vi "FindAdaptableTerm.vi"(0 "Adaptable Terms":cluster{"Type":T2, "Id":T1, "Broken":bool}[](array[cluster]), 1 "Id":string) -> (2 "Type":T2, 3 "Id out":T1, 4 "Found?":bool, 5 "Broken":bool)   [LabVIEW 2017]
uses:
  <vilib>/XNodeSupport/XNodeType.ctl
  <vilib>/XNodeSupport/XNodeString.ctl
  <vilib>/XNodeSupport/NI_XNodeSupport.lvlib
panel:
  # "LVHDF5 Toolkit\nCopyright (c) 2005-2013 by Jason D. Sommerville\nCopyright (c) 2014 by UPVI, LLC.\n\nThis use and distribution of this file is governed by the terms found in \nLICENSE.txt distributed with this toolkit and installed at\n <user.lib>\\_lvhdf5\\LICENSE.txt"
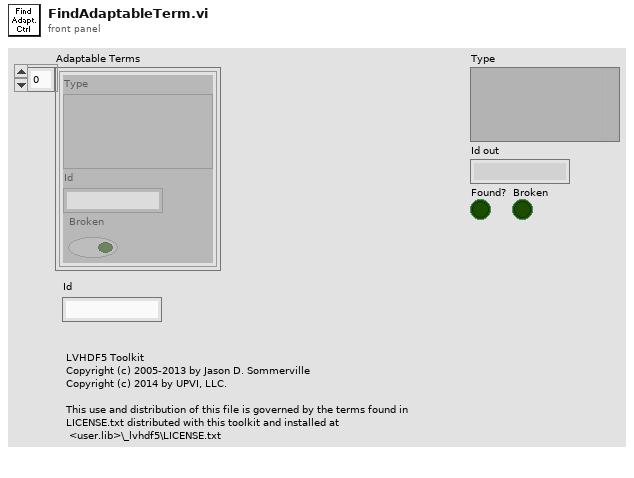
[diagram p1: front panel]
types:
  T1 = typedef "NI_XNodeSupport.lvlib/XNodeString.ctl" = string
  T2 = typedef "NI_XNodeSupport.lvlib/XNodeType.ctl" = variant
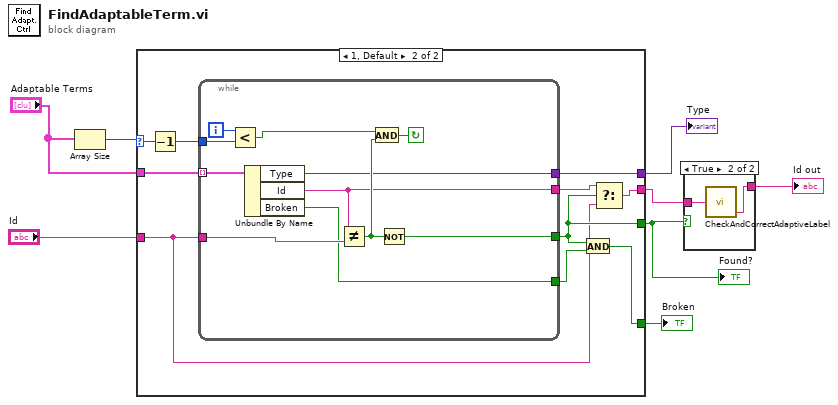
[diagram p0: block diagram]
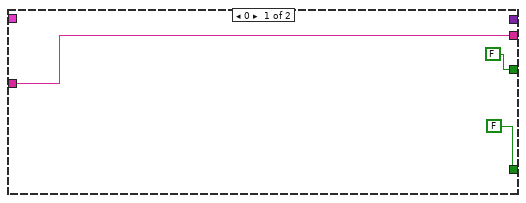
[diagram p3: hidden frame]
diagram:
  n1 = Array Size(array="Adaptable Terms") -> (size(s)=w8:i32)
  n2 = case shown="1, Default" w8 {
    selector: w8 -> [_ w20]
    tunnel: "Adaptable Terms" -> [_ w21]
    tunnel: "Id" -> [w10 w12]
    tunnel: [FALSE w13] -> w1
    tunnel: [w10 w14] -> w3
    tunnel: [_ w18] -> w5
    tunnel: [FALSE w16] -> w4
    frame 0 {
    }
    frame 1, Default {
      n3 = Decrement(x=w20) -> (x-1=w19:i32)
      n4 = while {
        tunnel: w21 -> [w30] mode=indexing
        tunnel: w19 -> [w31]
        tunnel: w12 -> [w29]
        tunnel: [w25] -> w13
        tunnel: [w24] -> w15
        tunnel: [w23] -> w18
        tunnel: [w22] -> w17
        i -> [w32]
        stop <- w27 continue-if-true
        n5 = Less?(x=w32, y=w31) -> (x < y?=w28:bool)
        n6 = Unbundle By Name(w30) -> ("Type"=w23:T2, "Id"=w24:T1, "Broken"=w22:bool)
        n7 = Not Equal?(x=w24, y=w29) -> (x != y?=w26:bool)
        n8 = And(x=w28, y=w26) -> (x .and. y?=w27:bool)
        n9 = Not(x=w26) -> (.not. x?=w25:bool)
      }
      n10 = And(x=w13, y=w17) -> (x .and. y?=w16:bool)
      n11 = Select(t=w15, s=w13, f=w12) -> (s? t:f=w14:T1)
    }
  }
  "Type" <- w5
  "Found?" <- w1
  "Broken" <- w4
  n12 = case shown="True" w1 {
    tunnel: w3 -> [w33 w35]
    tunnel: [w33 w34] -> w2
    frame False {
    }
    frame True {
      n13 = call <vilib>:"CheckAndCorrectAdaptiveLabel.vi"("Control Label"=w35) -> ("Corrected Control Label"=w34:string)  [unwired: 2 out]
    }
  }
  "Id out" <- w2
